vi "CRYUnflatten Recall.vi"(11 "Flatten Recall":string) -> (0 "Error?":bool=TRUE, 2 "Recall setup":T1={"Name"="Test for Signal [L]", "filepath"="Test for Signal [L]", "all or last"=0, "File Path Mode"=0, "Curve Names"=[], "format string"={"dB Format String out"="", "Lin Format String out"=""}, "Template"=[], "Axis"=0, "*.imp Path"=path "", "Filepath option"=0, "ML Value"=0.0, "user defined"="Test for Signal [L]", "Curves Selected?"=[], "Help"="", "Tab Value"=enum."Setting", "Selector"=0, "Use Default"=FALSE} {"Selector" items=["Space", "Underscores", "None"]; "Axis" scale=0.0..2.0; "Template" format="%#.0f"}, 3 "Header info":T2={"Data type"="Data            ", "Version"=1, "Dimensions"=0})   [LabVIEW 2013]
uses:
  Typedef Control/CRYRecall Cluster.ctl
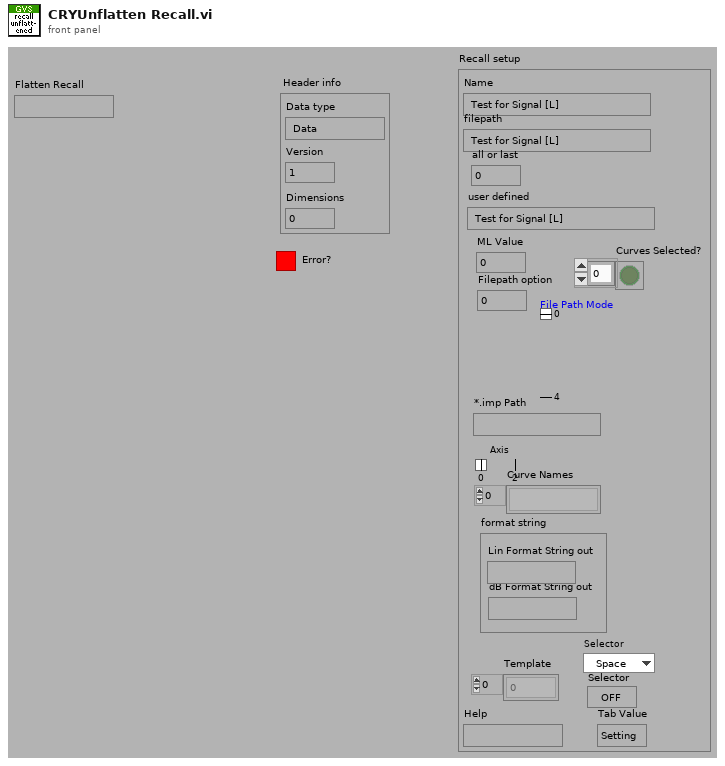
[diagram p1: front panel]
types:
  T1 = typedef "CRYRecall Cluster.ctl" = cluster{"Name":string, "filepath":string, "all or last":i32, "File Path Mode":u16, "Curve Names":string[], "format string":cluster{"dB Format String out":string, "Lin Format String out":string}, "Template":u16[], "Axis":u16, "*.imp Path":path, "Filepath option":i16, "ML Value":dbl, "user defined":string, "Curves Selected?":bool[], "Help":string, "Tab Value":enum32{"Setting", "Help"}, "Selector":i32, "Use Default":bool}
  T2 = cluster{"Data type":string, "Version":u16, "Dimensions":u8}
  T3 = cluster{"Name":string, "filepath":string, "all or last":i32, "File Path Mode":u16, "Curve Names":string[], "format string":cluster{"dB Format String out":string, "Lin Format String out":string}, "Template":u16[], "Axis":u16, "*.imp Path":path, "Filepath option":i16, "ML Value":dbl, "user defined":string, "Curves Selected?":bool[], "Help":string, "Tab Value":enum32{"Setting", "Help"}, "Selector":i32, "Use Default":bool}
  T4 = cluster{"Hide":string, "Precision":string, "Digits":string, "Notation":string}
  T5 = cluster{"unsigned byte array[0]":u8, "unsigned byte array[1]":u8, "unsigned byte array[2]":u8}
  T6 = cluster{"Name":string, "filepath":string, "all or last":i32, "File Path Mode":u16, "Curve Names":string[], "format string":cluster{"dB Format String out":string, "Lin Format String out":string}, "Template":u16[], "Axis":u16, "*.imp Path":path, "Filepath option":i16, "ML Value":dbl, "user defined":string, "Curves Selected?":bool[]}
  T7 = cluster{"dB Format String out":string, "Lin Format String out":string}
  T8 = cluster{"Name":string, "filepath":string, "all or last":i32, "File Path Mode":u16, "Curve Names":string[], "format string":cluster{"dB Format String out":string, "Lin Format String out":string}, "Template":u16[], "Axis":u16, "*.imp Path":path, "Filepath option":i16, "ML Value":dbl, "user defined":string, "Curves Selected?":bool[], "Help":string, "Tab Value":enum32{"Setting", "Help"}}
  T9 = cluster{"substring":string, u16, "unsigned byte array[2]":u8}
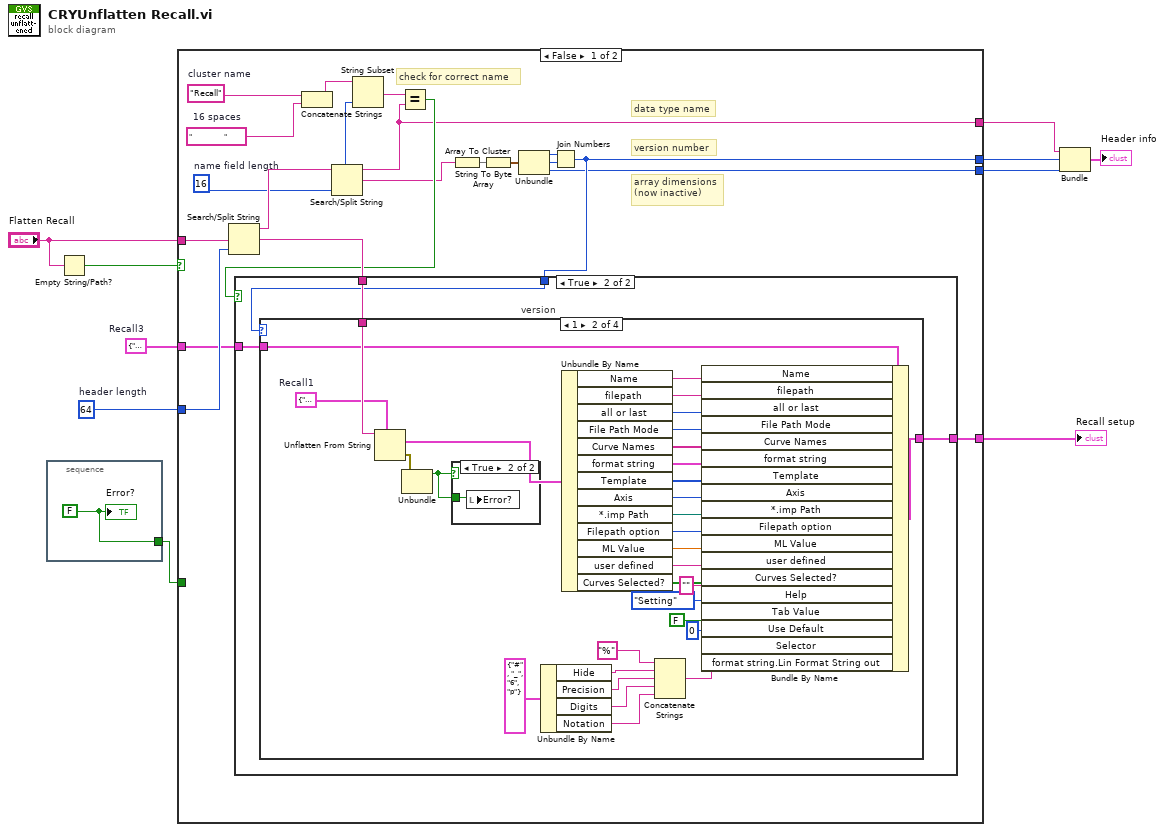
[diagram p0: block diagram]
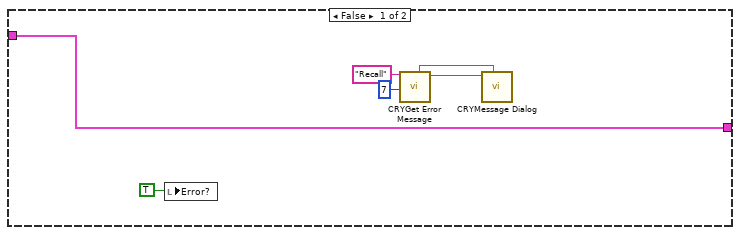
[diagram p2: hidden frame]
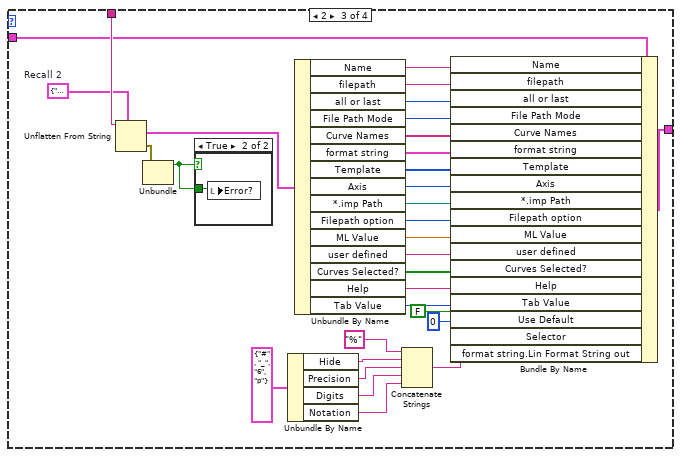
[diagram p5: hidden frame]
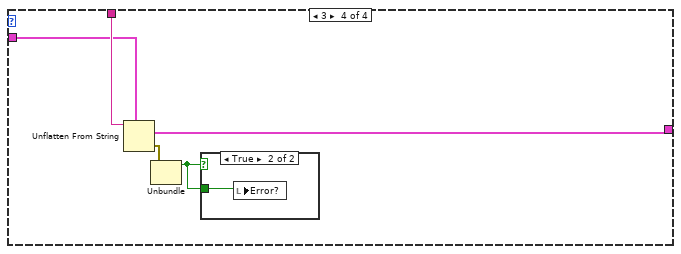
[diagram p7: hidden frame]
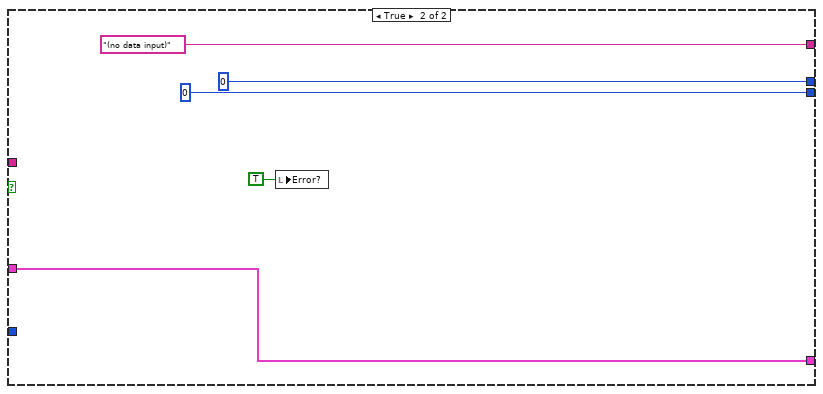
[diagram p9: hidden frame]
diagram:
  w2 = T3 {"Name"="Test for Signal [L]", "filepath"="Test for Signal [L]", "all or last"=0, "File Path Mode"=0, "Curve Names"=[], "format string"={"dB Format String out"="", "Lin Format String out"=""}, "Template"=[], "Axis"=0, "*.imp Path"=path "", "Filepath option"=0, "ML Value"=0.0, "user defined"="Test for Signal [L]", "Curves Selected?"=[], "Help"="", "Tab Value"=enum."Setting", "Selector"=0, "Use Default"=FALSE}  # Recall3
  w8 = 64  # header length
  n1 = stacked-sequence {
    tunnel: [w11] -> w3
    frame #0 {
      w11 = FALSE
      "Error?" <- w11
    }
  }
  n2 = Empty String/Path?(string/path="Flatten Recall") -> (empty?=w9:bool)
  n3 = case shown="False" w9 {
    tunnel: "Flatten Recall" -> [w31 _]
    tunnel: w8 -> [w25 _]
    tunnel: [w22 u16 0] -> w6
    tunnel: [w14 u8 0] -> w7
    tunnel: [w15 "(no data input)" ("substring")] -> w5
    tunnel: w3 -> [_ _]
    tunnel: [w13 w113] -> w1
    tunnel: w2 -> [w12 w113]
    frame False {
      w19 = "                "  # 16 spaces
      w20 = "Recall"  # cluster name
      w17 = 16  # name field length
      # "check for correct name"
      # "array dimensions\n(now inactive)"
      # "version number"
      # "data type name"
      n4 = Search/Split String(string=w31, offset (0)=w25) -> (substring before match=w24:string, match + rest of string=w26:string)  [unwired: 2 out]
      n5 = Concatenate Strings(w20, w19) -> (w18:string)
      n6 = Search/Split String(string=w24, offset (0)=w17) -> (substring before match=w15:string, match + rest of string=w21:string)  [unwired: 2 out]
      n7 = String Subset(string=w18, length (rest)=w17) -> (substring=w16:string)  [unwired: 1 out]
      n8 = Equal?(x=w16, y=w15) -> (x = y?=w23:bool)
      n9 = String To Byte Array(string=w21) -> (unsigned byte array=w30:u8[])
      n10 = Array To Cluster(array=w30) -> (cluster=w29:T5)
      n11 = Unbundle(w29) -> ("unsigned byte array[0]"=w28:u8, "unsigned byte array[1]"=w27:u8, "unsigned byte array[2]"=w14:u8)
      n12 = Join Numbers(hi=w28, lo=w27) -> ((hi.lo)=w22:u16)
      n13 = case shown="True" w23 {
        tunnel: w26 -> [_ w41]
        tunnel: w22 -> [_ w40]
        tunnel: [w36 w39] -> w13
        tunnel: w12 -> [w36 w38]
        frame False {
          n14 = local write "Error?"(TRUE) -> ()
          n15 = call "CRYGet Error Message.vi"("Error No"=7 ("No"), "Kind"="Recall") -> ("Message"=w33:string, "Window Title"=w32:string)  [unwired: 4 in, 4 out]
          n16 = call "CRYMessage Dialog.vi"("Window Title"=w32, "Message Content"=w33) -> ()  [unwired: 8 in, 2 out]
        }
        frame True {
          n17 = case "version" shown="1" w40 {
            tunnel: w41 -> [_ w73 w105 w111]
            tunnel: [w42 w68 w101 w107] -> w39
            tunnel: w38 -> [w42 w67 w100 w108]
            frame Default {
            }
            frame 1 {
              w70 = T6 {"Name"="", "filepath"="", "all or last"=0, "File Path Mode"=0, "Curve Names"=[], "format string"={"dB Format String out"="", "Lin Format String out"=""}, "Template"=[], "Axis"=0, "*.imp Path"=path "", "Filepath option"=0, "ML Value"=0.0, "user defined"="", "Curves Selected?"=[]}  # Recall1
              n18 = Unflatten From String(type=w70, binary string=w73) -> (value=w69:T6, error out=w71:errorcluster)  [unwired: 1 in, 3 out]
              n19 = Unbundle(w71) -> ("status"=w72:bool)  [unwired: 2 out]
              n20 = case shown="True" w72 {
                tunnel: w72 -> [_ w74]
                frame False {
                }
                frame True {
                  n21 = local write "Error?"(w74) -> ()
                }
              }
              n22 = Unbundle By Name(T4 {"Hide"="#", "Precision"="_", "Digits"="6", "Notation"="p"} ("Num format")) -> ("Hide"=w49:string, "Precision"=w48:string, "Digits"=w47:string, "Notation"=w46:string)
              n23 = Unbundle By Name(w69) -> ("Name"=w66:string, "filepath"=w65:string, "all or last"=w64:i32, "File Path Mode"=w63:u16, "Curve Names"=w62:string[], "format string"=w61:T7, "Template"=w60:u16[], "Axis"=w59:u16, "*.imp Path"=w58:path, "Filepath option"=w57:i16, "ML Value"=w56:dbl, "user defined"=w55:string, "Curves Selected?"=w54:bool[])
              n24 = Concatenate Strings("%" ("string"), w49, w48, w47, w46) -> (w43:string)
              n25 = Bundle By Name(cluster=w67, "Name"=w66, "filepath"=w65, "all or last"=w64, "File Path Mode"=w63, "Curve Names"=w62, "format string"=w61, "Template"=w60, "Axis"=w59, "*.imp Path"=w58, "Filepath option"=w57, "ML Value"=w56, "user defined"=w55, "Curves Selected?"=w54, "Help"="", "Tab Value"=enum32{"Setting", "Help"}."Setting", "Use Default"=FALSE, "Selector"=0, "format string.Lin Format String out"=w43) -> (w68:T3)
            }
            frame 2 {
              w83 = T8 {"Name"="Test for Signal [L]", "filepath"="Test for Signal [L]", "all or last"=0, "File Path Mode"=0, "Curve Names"=[], "format string"={"dB Format String out"="", "Lin Format String out"=""}, "Template"=[], "Axis"=0, "*.imp Path"=path "", "Filepath option"=0, "ML Value"=0.0, "user defined"="Test for Signal [L]", "Curves Selected?"=[], "Help"="", "Tab Value"=enum."Setting"}  # Recall 2
              n26 = Unflatten From String(type=w83, binary string=w105) -> (value=w102:T8, error out=w103:errorcluster)  [unwired: 1 in, 3 out]
              n27 = Unbundle(w103) -> ("status"=w104:bool)  [unwired: 2 out]
              n28 = case shown="True" w104 {
                tunnel: w104 -> [_ w106]
                frame False {
                }
                frame True {
                  n29 = local write "Error?"(w106) -> ()
                }
              }
              n30 = Unbundle By Name(T4 {"Hide"="#", "Precision"="_", "Digits"="6", "Notation"="p"} ("Num format")) -> ("Hide"=w81:string, "Precision"=w80:string, "Digits"=w79:string, "Notation"=w78:string)
              n31 = Unbundle By Name(w102) -> ("Name"=w95:string, "filepath"=w94:string, "all or last"=w93:i32, "File Path Mode"=w92:u16, "Curve Names"=w91:string[], "format string"=w90:T7, "Template"=w89:u16[], "Axis"=w88:u16, "*.imp Path"=w87:path, "Filepath option"=w86:i16, "ML Value"=w99:dbl, "user defined"=w98:string, "Curves Selected?"=w97:bool[], "Help"=w85:string, "Tab Value"=w84:enum32{"Setting", "Help"})
              n32 = Concatenate Strings("%" ("string"), w81, w80, w79, w78) -> (w75:string)
              n33 = Bundle By Name(cluster=w100, "Name"=w95, "filepath"=w94, "all or last"=w93, "File Path Mode"=w92, "Curve Names"=w91, "format string"=w90, "Template"=w89, "Axis"=w88, "*.imp Path"=w87, "Filepath option"=w86, "ML Value"=w99, "user defined"=w98, "Curves Selected?"=w97, "Help"=w85, "Tab Value"=w84, "Use Default"=FALSE, "Selector"=0, "format string.Lin Format String out"=w75) -> (w101:T3)
            }
            frame 3 {
              n34 = Unflatten From String(type=w108, binary string=w111) -> (value=w107:T3, error out=w109:errorcluster)  [unwired: 1 in, 3 out]
              n35 = Unbundle(w109) -> ("status"=w110:bool)  [unwired: 2 out]
              n36 = case shown="True" w110 {
                tunnel: w110 -> [_ w112]
                frame False {
                }
                frame True {
                  n37 = local write "Error?"(w112) -> ()
                }
              }
            }
          }
        }
      }
    }
    frame True {
      n38 = local write "Error?"(TRUE ("Error?")) -> ()
    }
  }
  "Recall setup" <- w1
  n39 = Bundle("substring"=w5, w6, "unsigned byte array[2]"=w7) -> (→"Header info":T9)  [unwired: 1 out]
